vi "SignalReceiver.GlobalSignalReceData.vi"(8 "error in (no error)":errorcluster, 11 "SignalReceiver":refnum<class "SignalReceiver.lvclass">) -> (0 "error out":errorcluster, 3 "SignalReceiver out":refnum<class "SignalReceiver.lvclass">)   [LabVIEW 2020, in "SignalReceiver.lvclass"]
doc: "---------------------------------------------------------------\nJKI State Machine Objects™\nhttp://jki.net/state-machine-objects/\nCopyright (C) 2005-2015, JKI <info@jki.net>\nALL RIGHTS RESERVEDJKI State Machine Objects (SMO) 1.0.0.5\nJKI - JKI\nCopyright (c) 2016, JKI"
uses:
  SignalReceiver.lvclass
  GlobalData_operation.ctl
panel:
  out "SignalDatOut":dbl[][](array[numeric])
  in  "SignalDatIn":dbl[][](array[numeric])
  out "Update":bool
  in  "operation":T1
  # "For instructions on how to use the JKI State Machine Objects, examples and video tutorials, visit:\nhttp://jki.net/state-machine-objects/\n\nJKI State Machine Objects™\nhttp://jki.net/state-machine-objects/\nCopyright (C) 2005-2015, JKI <info@jki.net>\nALL RIGHTS RESERVED"
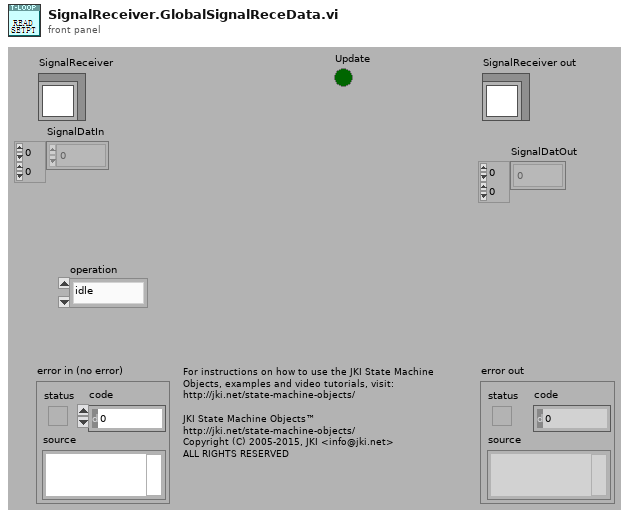
[diagram p1: front panel]
types:
  T1 = typedef "GlobalData_operation.ctl" = enum16{"idle", "read", "write", "clear", "init", "destroy"}
  T2 = typedef "SignalReceiver.lvclass/PrivateData--Ref.ctl" = refnum<data-value>
  T3 = typedef "SignalReceiver.lvclass/PrivateData--Cluster.ctl" = cluster{"Public Events":T4, "Private Events":T5, "SignalArrySelect":T6, "SignalDataReciArry":T7}
  T4 = typedef "SignalReceiver.lvclass/PublicEvents--Cluster.ctl" = cluster{"Setpoint Changed":refnum<user-event>, "Value Changed":refnum<user-event>}
  T5 = typedef "SignalReceiver.lvclass/PrivateEvents--Cluster.ctl" = cluster{"AsyncMethod":refnum<user-event>, "Start_Stop":refnum<user-event>}
  T6 = typedef "SignalReceiver.lvclass/SignalArrySelecte.ctl" = cluster{"Port_No.":refnum<k21>, "XNET Signal":refnum<k21>[]}
  T7 = typedef "SignalReceiver.lvclass/SignalDataArry.ctl" = cluster{"SignalDataReceiveArry":dbl[][], "Update":bool}
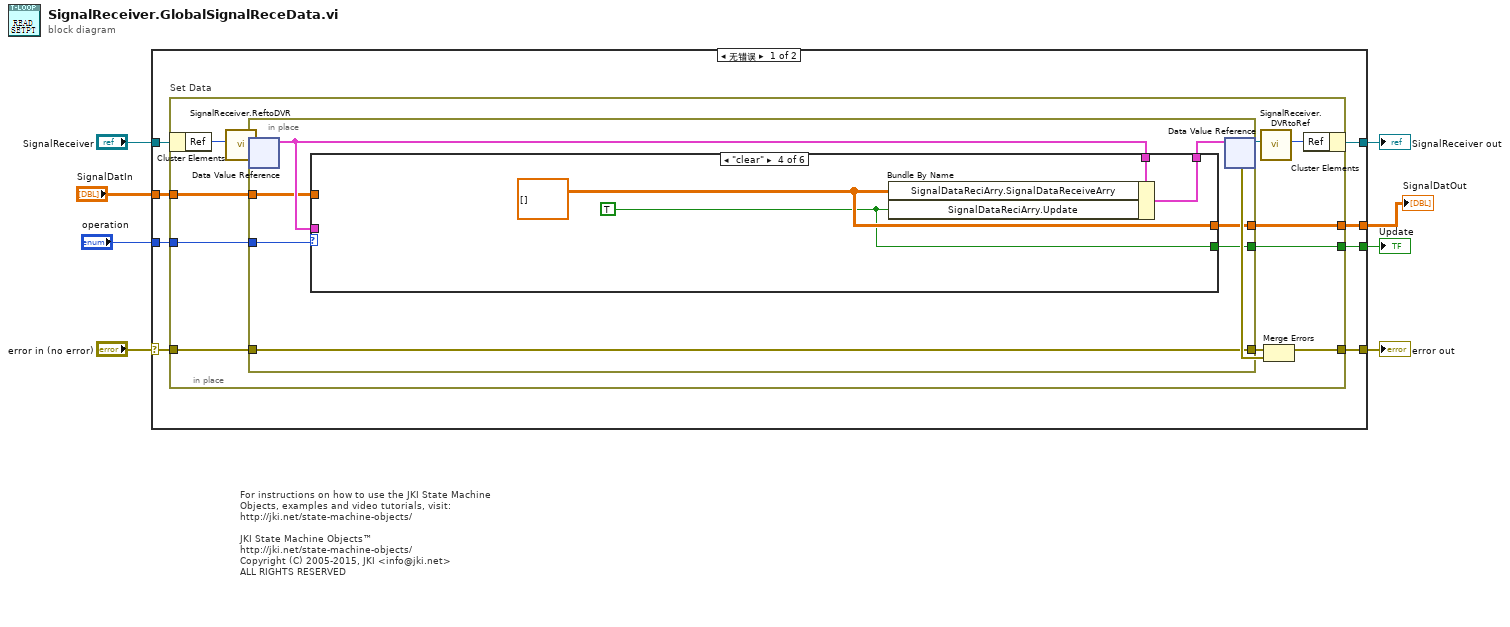
[diagram p0: block diagram]
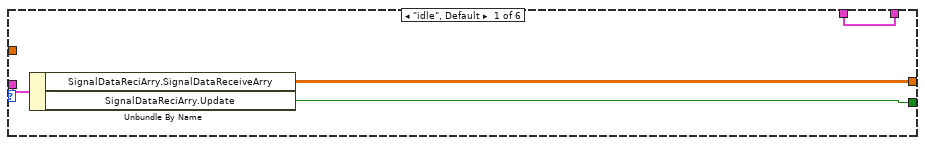
[diagram p2: hidden frame]
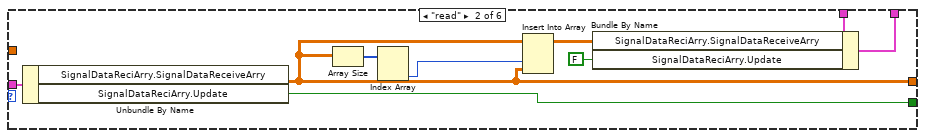
[diagram p3: hidden frame]
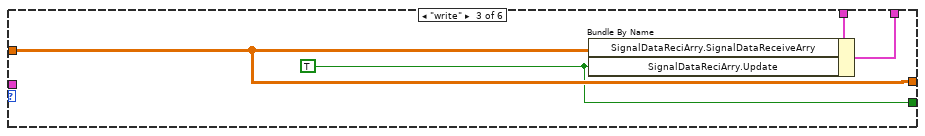
[diagram p4: hidden frame]
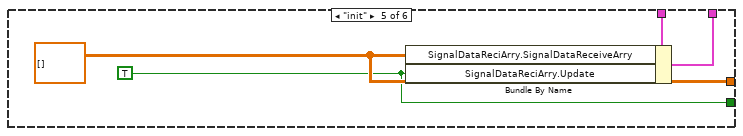
[diagram p5: hidden frame]
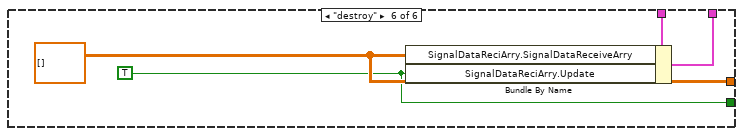
[diagram p6: hidden frame]
diagram:
  # "For instructions on how to use the JKI State Machine Objects, examples and video tutorials, visit:\nhttp://jki.net/state-machine-objects/\n\nJKI State Machine Objects™\nhttp://jki.net/state-machine-objects/\nCopyright (C) 2005-2015, JKI <info@jki.net>\nALL RIGHTS RESERVED"
  n1 = case shown="无错误" "error in (no error)" {
    selector: "error in (no error)" -> [w15 w65]
    tunnel: "SignalReceiver" -> [w16 w66]
    tunnel: [w14 w65] -> w7
    tunnel: [w13 w66] -> w6
    tunnel: [w12 _] -> w1
    tunnel: "operation" -> [w11 _]
    tunnel: [w10 _] -> w3
    tunnel: "SignalDatIn" -> [w9 _]
    frame No Error {
      n2 = in-place "Set Data" {
        in-place-border: w15 -> [w28]
        in-place-border: [w25] -> w14
        in-place-border: [w20] -> w12
        in-place-border: w11 -> [w19]
        in-place-border: [w18] -> w10
        in-place-border: w9 -> [w17]
        n3 = in-place-cluster #1(w16) -> ("Ref"=w24:u32)
        n4 = call "SignalReceiver.ReftoDVR.vi"("Ref"=w24) -> ("Ref"=w23:T2)  [unwired: 10 in]
        n5 = in-place {
          in-place-border: w28 -> [w35]
          in-place-border: [w35] -> w26
          in-place-border: [w34] -> w20
          in-place-border: w19 -> [w33]
          in-place-border: [w32] -> w18
          in-place-border: w17 -> [w29]
          n6 = in-place-dvr #2(w23) -> (w31:T3)  [unwired: 1 out]
          n7 = case shown="\"clear\"" w33 {
            tunnel: [w38 w41 w50 w54 w58 w62] -> w34
            tunnel: w31 -> [w39 w48 _ _ _ _]
            tunnel: [w37 w47 w49 w53 w57 w61] -> w32
            tunnel: w31 -> [w36 w46 w52 w56 w60 w64]
            tunnel: [w36 w45 w51 w55 w59 w63] -> w30
            tunnel: w29 -> [_ _ w50 _ _ _]
            frame "idle", Default {
              n8 = Unbundle By Name(w39) -> ("SignalDataReciArry.SignalDataReceiveArry"=w38:dbl[][], "SignalDataReciArry.Update"=w37:bool)
            }
            frame "read" {
              n9 = Unbundle By Name(w48) -> ("SignalDataReciArry.SignalDataReceiveArry"=w41:dbl[][], "SignalDataReciArry.Update"=w47:bool)
              n10 = Array Size(array=w41) -> (size(s)=w43:i32[])
              n11 = Index Array(array=w43) -> (element #2=w42:i32)  [unwired: 2 in, 1 out]
              n12 = Insert Into Array(array=w41, index (col)=w42, new element=w41) -> (w40:dbl[][])  [unwired: 1 in]
              n13 = Bundle By Name(cluster=w46, "SignalDataReciArry.SignalDataReceiveArry"=w40, "SignalDataReciArry.Update"=FALSE) -> (w45:T3)
            }
            frame "write" {
              w49 = TRUE ("SignalDataReciArry.Update")
              n14 = Bundle By Name(cluster=w52, "SignalDataReciArry.SignalDataReceiveArry"=w50, "SignalDataReciArry.Update"=w49) -> (w51:T3)
            }
            frame "clear" {
              w54 = dbl[][] [] ("SignalDataReciArry.SignalDataReceiveArry")
              w53 = TRUE ("SignalDataReciArry.Update")
              n15 = Bundle By Name(cluster=w56, "SignalDataReciArry.SignalDataReceiveArry"=w54, "SignalDataReciArry.Update"=w53) -> (w55:T3)
            }
            frame "init" {
              w58 = dbl[][] [] ("SignalDataReciArry.SignalDataReceiveArry")
              w57 = TRUE ("SignalDataReciArry.Update")
              n16 = Bundle By Name(cluster=w60, "SignalDataReciArry.SignalDataReceiveArry"=w58, "SignalDataReciArry.Update"=w57) -> (w59:T3)
            }
            frame "destroy" {
              w62 = dbl[][] [] ("SignalDataReciArry.SignalDataReceiveArry")
              w61 = TRUE ("SignalDataReciArry.Update")
              n17 = Bundle By Name(cluster=w64, "SignalDataReciArry.SignalDataReceiveArry"=w62, "SignalDataReciArry.Update"=w61) -> (w63:T3)
            }
          }
          n18 = in-place-dvr #2(w30) -> (w22:T2, w27:errorcluster)
        }
        n19 = call "SignalReceiver.DVRtoRef.vi"("Ref"=w22) -> ("Ref"=w21:u32)  [unwired: 10 in]
        n20 = Merge Errors(w26, w27) -> (w25:errorcluster)
        n21 = in-place-cluster #1("Ref"=w21) -> (w13:refnum<class "SignalReceiver.lvclass">)
      }
    }
    frame Error {
    }
  }
  "error out" <- w7
  "SignalReceiver out" <- w6
  "Update" <- w3
  "SignalDatOut" <- w1
